vi "Begin.vi"(8 "error in":errorcluster) -> (0 "error out":errorcluster)   [LabVIEW 2018]
doc: "Called before other user functions, this VI is expected to open initial I/O refnums, load in file data, and do all program initialization. Notice that the <B>error out</B> terminal is simply used for data flow. Wiring it to other structures or subVIs ensures that this VI runs first."
uses:
  <vilib>/Rock Robotics/WPI/Joystick/WPI_JoystickDeviceEnum.ctl
  <vilib>/Rock Robotics/WPI/DriverStation/WPI_DriverStationRobotMode2.ctl
  <vilib>/Rock Robotics/SystemInterfaces/DIO/FPGA_DIOChannel.ctl
  <vilib>/Rock Robotics/WPI/Solenoid/WPI_SolenoidChannel.ctl
  <vilib>/Rock Robotics/WPI/ThirdParty/Phoenix-LabVIEW/Motor Controller/Controls/CTRE_Phoenix_MotorControl_NeutralMode.ctl
  Robot Global Data.vi
  <vilib>/Rock Robotics/Network Tables/NT Write String Array.vi
  <vilib>/Rock Robotics/WPI/Solenoid/WPI_SolenoidOpenDouble.vi
  <vilib>/Rock Robotics/WPI/RobotDrive/WPI_RobotDriveOpen2MotorWithExistingMotors.vi
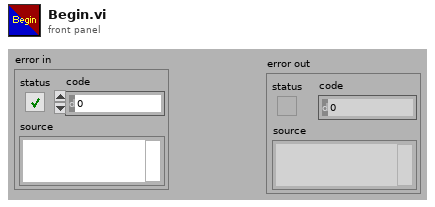
[diagram p1: front panel]
types:
  T1 = typedef "WPI_JoystickDeviceEnum.ctl" = enum16{"USB 0", "USB 1", "USB 2", "USB 3", "USB 4", "USB 5"}
  T2 = typedef "FPGA_DIOChannel.ctl" = enum8{"DIO 0", "DIO 1", "DIO 2", "DIO 3", "DIO 4", "DIO 5", "DIO 6", "DIO 7", "DIO 8", "DIO 9", "DIO MXP 0", "DIO MXP 1", "DIO MXP 2", "DIO MXP 3", "DIO MXP 4", "DIO MXP 5", "DIO MXP 6", "DIO MXP 7", "DIO MXP 8", "DIO MXP 9", "DIO MXP 10", "DIO MXP 11", "DIO MXP 12", "DIO MXP 13", "DIO MXP 14", "DIO MXP 15", "SPI Port CS1", "SPI Port CS2", "SPI Port CS3", "SPI Port MISO", "SPI Port MOSI", "Invalid"}
  T3 = typedef "WPI_SolenoidChannel.ctl" = enum8{"Solenoid 0", "Solenoid 1", "Solenoid 2", "Solenoid 3", "Solenoid 4", "Solenoid 5", "Solenoid 6", "Solenoid 7", "Invalid"}
  T4 = typedef "WPI_DriverStationRobotMode2.ctl" = enum16{"Autonomous Disabled", "Autonomous Enabled", "Teleop Disabled", "Teleop Enabled", "Disconnected", "Finish", "Test Disabled", "Test Enabled", "Emergency Stopped"}
  T5 = cluster{"proportional gain (Kc)":dbl, "integral time (Ti, min)":dbl, "derivative time (Td, min)":dbl}
  T6 = typedef "WPI_JoystickDevRef.ctl" = cluster{"Device":T1}
  T7 = typedef "CTRE_Phoenix_MotorControl_NeutralMode.ctl" = enum8{"EEPROMSetting", "Override to Coast", "Override to Brake"}
  T8 = cluster{"Yaw":dbl, "Roll":dbl, "Pitch":dbl, "Heading":dbl, "Fused Heading":dbl}
  T9 = typedef "WPI_MotorControlDeviceRef.ctl" = cluster{"DeviceStatus":errorcluster, "Type":T10, "PWM":cluster{"PWM Channel":T11, "DeadBand":T12}, "CAN":cluster{"Device Number":u8, "SetOutput VI Ref":variant, "GetOutput VI Ref":variant, "Enable VI Ref":variant, "Disable VI Ref":variant, "Data":variant}, "Invert":bool, "DIO PWM":cluster{"PWM \"Enable\" Channel":T11, "DIOChannel":T2, "PWM Rate":dbl}}
  T10 = typedef "WPI_MotorControlType.ctl" = enum16{"PWM", "CAN", "DIO PWM"}
  T11 = typedef "FPGA_DIOPWMChannel.ctl" = enum8{"PWM 0", "PWM 1", "PWM 2", "PWM 3", "PWM 4", "PWM 5", "PWM 6", "PWM 7", "PWM 8", "PWM 9", "PWM MXP 0", "PWM MXP 1", "PWM MXP 2", "PWM MXP 3", "PWM MXP 4", "PWM MXP 5", "PWM MXP 6", "PWM MXP 7", "PWM MXP 8", "PWM MXP 9", "Invalid"}
  T12 = typedef "WPI_PWMDeadband.ctl" = cluster{"Name":string, "maxPositivePwm":i32, "minPositivePwm":i32, "centerPwm":i32, "maxNegativePwm":i32, "minNegativePwm":i32, "angularRange":u16}
  T13 = typedef "WPI_RobotDriveDevRef.ctl" = cluster{"DevStatus":errorcluster, "Motors[]":T9[], "Square Inputs":bool, "Max Output":dbl}
  T14 = typedef "WPI_DigitalInputDevRef.ctl" = cluster{"DevStatus":errorcluster, "DIO Channel":T2}
  T15 = typedef "WPI_SolenoidDevRef.ctl" = cluster{"DevStatus":errorcluster, "Pneumatics Control Module":u8, "Forward Solenoid Channel":T3, "Reverse Solenoid Channel":T3}
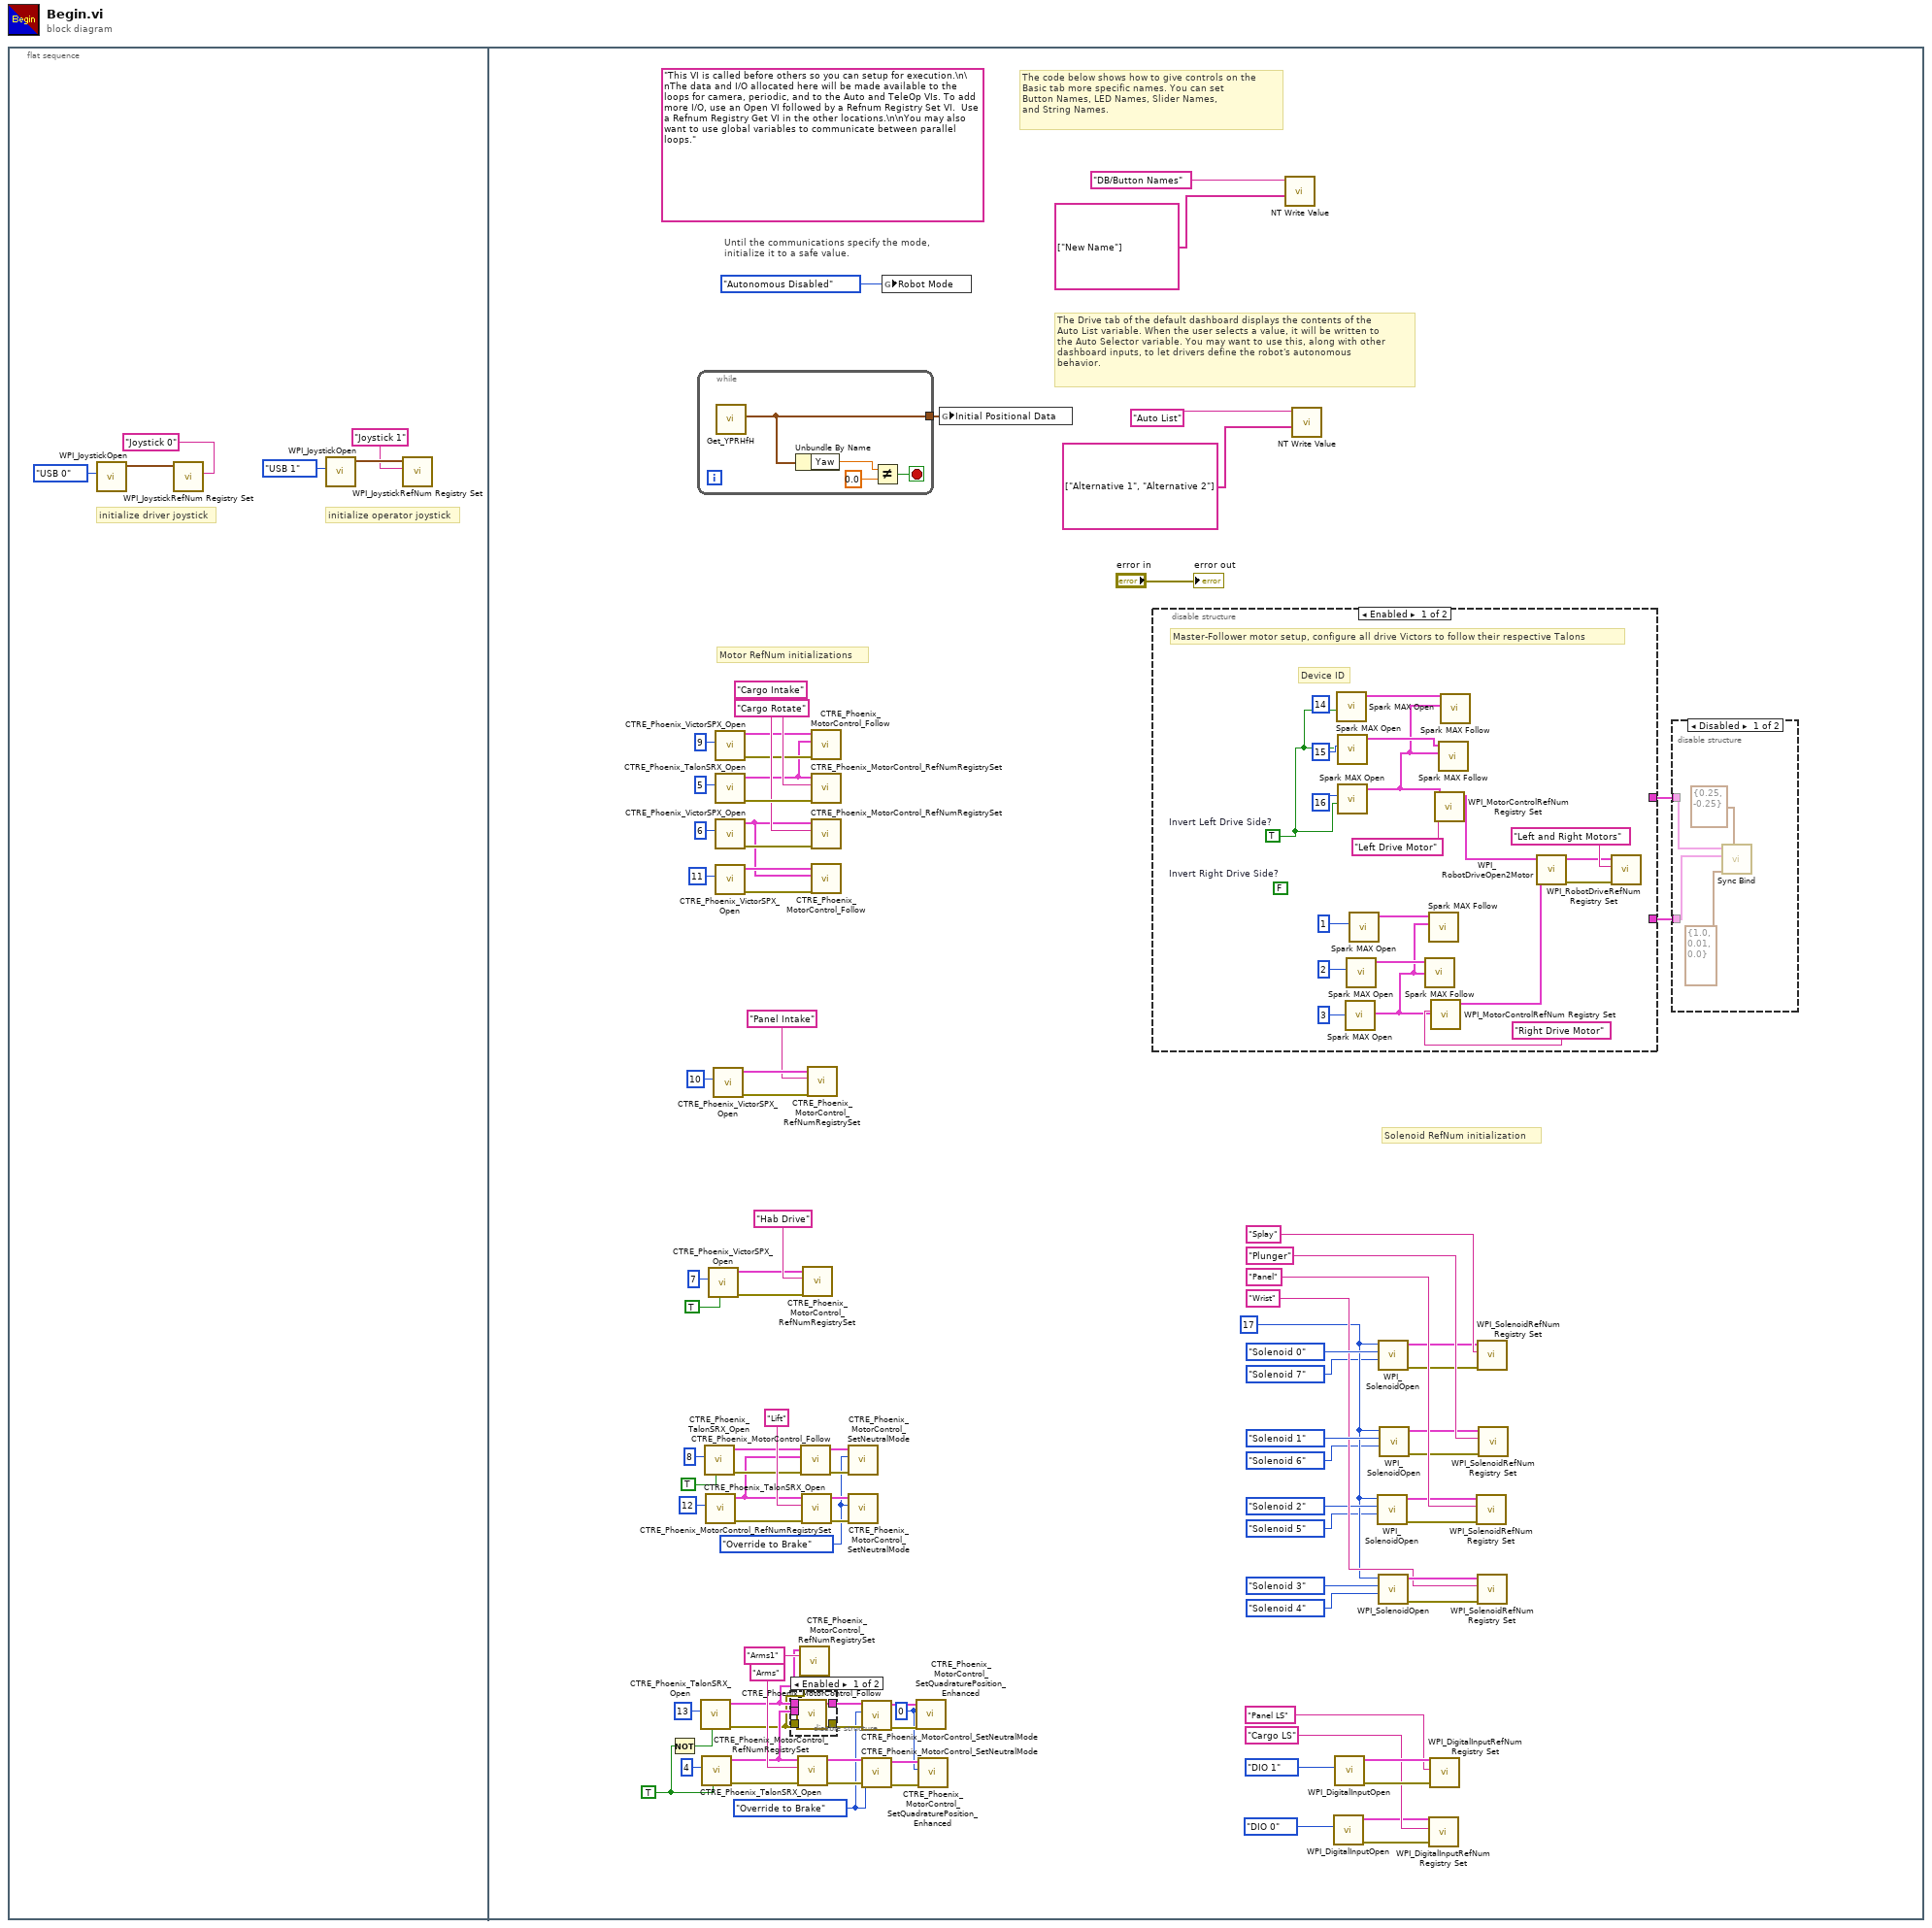
[diagram p0: block diagram]
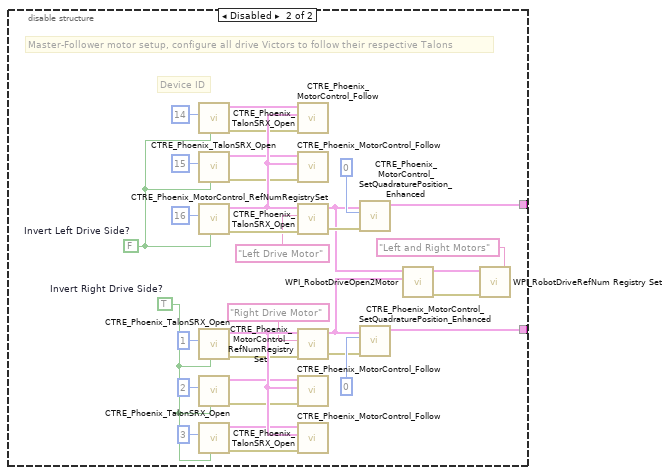
[diagram p4: hidden frame]
diagram:
  n1 = flat-sequence {
    frame #0 {
      # "initialize operator joystick"
      # "initialize driver joystick"
      n2 = call <vilib>:"WPI_JoystickOpen.vi"("JoystickDevice"=WPI_JoystickDeviceEnum."USB 0") -> ("JoystickDevRef"=w5:T6)  [unwired: 10 in]
      n3 = call <vilib>:"WPI_JoystickRefNum Registry Set.vi"("refnum name"="Joystick 0", "JoystickDevRef"=w5) -> ()  [unwired: 8 in, 2 out]
      n4 = call <vilib>:"WPI_JoystickOpen.vi"("JoystickDevice"=WPI_JoystickDeviceEnum."USB 1") -> ("JoystickDevRef"=w6:T6)  [unwired: 10 in]
      n5 = call <vilib>:"WPI_JoystickRefNum Registry Set.vi"("refnum name"="Joystick 1", "JoystickDevRef"=w6) -> ()  [unwired: 8 in, 2 out]
    }
    frame #1 {
      w8 = 0 ("New Position")
      w28 = u8 17 ("Pneumatics Control Module (0)")
      w34 = TRUE ("Invert")
      w36 = CTRE_Phoenix_MotorControl_NeutralMode."Override to Brake" ("Motor Control Neutral Mode")
      w42 = CTRE_Phoenix_MotorControl_NeutralMode."Override to Brake" ("Motor Control Neutral Mode")
      (unwired) "This VI is called before others so you can setup for execution.\n\nThe data and I/O allocated here will be made available to the loops for camera, periodic, and to the Auto and TeleOp VIs. To add more I/O, use an Open VI followed by a Refnum Registry Set VI.  Use a Refnum Registry Get VI in the other locations.\n\nYou may also want to use global variables to communicate between parallel loops."
      # "Motor RefNum initializations"
      # "Solenoid RefNum initialization"
      # "The Drive tab of the default dashboard displays the contents of the\nAuto List variable. When the user selects a value, it will be written to\nthe Auto Selector variable. You may want to use this, along with other\ndashboard inputs, to let drivers define the robot's autonomous\nbehavior."
      # "The code below shows how to give controls on the\nBasic tab more specific names. You can set\nButton Names, LED Names, Slider Names,\nand String Names."
      # "Until the communications specify the mode,\ninitialize it to a safe value."
      n6 = Not(x=w34) -> (.not. x?=w33:bool)
      n7 = while {
        tunnel: [w112] -> w27
        stop <- w113 stop-if-true
        n8 = call <vilib>:"Get_YPRHfH.vi"() -> ("YRPHfH"=w112:T8)  [unwired: 11 in]
        n9 = Unbundle By Name(w112) -> ("Yaw"=w114:dbl)
        n10 = Not Equal?(x=w114, y=0.0) -> (x != y?=w113:bool)
      }
      n11 = call <vilib>:"CTRE_Phoenix_TalonSRX_Open.vi"("Invert"=w33, "Device Number"=u8 13) -> ("error out"=w14:errorcluster, "CAN Talon SRX Ref"=w15:T9)  [unwired: 8 in]
      n12 = call <vilib>:"CTRE_Phoenix_TalonSRX_Open.vi"("Invert"=w34, "Device Number"=u8 4) -> ("error out"=w56:errorcluster, "CAN Talon SRX Ref"=w41:T9)  [unwired: 8 in]
      n13 = call <vilib>:"CTRE_Phoenix_TalonSRX_Open.vi"("Invert"=TRUE, "Device Number"=u8 8) -> ("error out"=w59:errorcluster, "CAN Talon SRX Ref"=w60:T9)  [unwired: 8 in]
      n14 = call <vilib>:"CTRE_Phoenix_TalonSRX_Open.vi"("Device Number"=u8 12) -> ("error out"=w58:errorcluster, "CAN Talon SRX Ref"=w57:T9)  [unwired: 9 in]
      n15 = call <vilib>:"CTRE_Phoenix_VictorSPX_Open.vi"("Invert"=TRUE, "Device Number"=u8 7) -> ("error out"=w50:errorcluster, "CAN Talon SRX Ref"=w49:T9)  [unwired: 8 in]
      n16 = call <vilib>:"CTRE_Phoenix_VictorSPX_Open.vi"("Device Number"=u8 10) -> ("error out"=w69:errorcluster, "CAN Talon SRX Ref"=w70:T9)  [unwired: 9 in]
      n17 = call <vilib>:"CTRE_Phoenix_VictorSPX_Open.vi"("Device Number"=u8 9) -> ("error out"=w18:errorcluster, "CAN Talon SRX Ref"=w19:T9)  [unwired: 9 in]
      n18 = call <vilib>:"CTRE_Phoenix_TalonSRX_Open.vi"("Device Number"=u8 5) -> ("error out"=w74:errorcluster, "CAN Talon SRX Ref"=w17:T9)  [unwired: 9 in]
      n19 = call <vilib>:"CTRE_Phoenix_VictorSPX_Open.vi"("Device Number"=u8 6) -> ("error out"=w73:errorcluster, "CAN Talon SRX Ref"=w46:T9)  [unwired: 9 in]
      n20 = call <vilib>:"CTRE_Phoenix_VictorSPX_Open.vi"("Device Number"=u8 11) -> ("error out"=w47:errorcluster, "CAN Talon SRX Ref"=w48:T9)  [unwired: 9 in]
      n21 = disable-structure shown="Enabled" {
        disable-tunnel: [w105 w107] -> w13
        disable-tunnel: [w104 w106] -> w45
        disable-tunnel: w41 -> [w103 _]
        disable-tunnel: w15 -> [w102 w107]
        disable-tunnel: w14 -> [w101 w106]
        frame Enabled {
          n22 = call <vilib>:"CTRE_Phoenix_MotorControl_Follow.vi"("error in (no error)"=w101, "Master Controller to Follow"=w103, "PhoenixMotorControlDevRef"=w102) -> ("error out"=w104:errorcluster, "PhoenixMotorControlDevRef"=w105:T9)  [unwired: 7 in]
        }
        frame Disabled {
        }
      }
      n23 = call <vilib>:"CTRE_Phoenix_MotorControl_RefNumRegistrySet.vi"("error in (no error)"=w56, "refnum name"="Arms", "PhoenixMotorControlDevRef"=w41) -> ("error out"=w44:errorcluster, "PhoenixMotorControlDevRef"=w43:T9)  [unwired: 7 in]
      n24 = call <vilib>:"CTRE_Phoenix_MotorControl_RefNumRegistrySet.vi"("error in (no error)"=w14, "refnum name"="Arms1", "PhoenixMotorControlDevRef"=w15) -> ()  [unwired: 7 in, 2 out]
      n25 = call <vilib>:"CTRE_Phoenix_MotorControl_Follow.vi"("error in (no error)"=w59, "Master Controller to Follow"=w57, "PhoenixMotorControlDevRef"=w60) -> ("error out"=w37:errorcluster, "PhoenixMotorControlDevRef"=w38:T9)  [unwired: 7 in]
      n26 = call <vilib>:"CTRE_Phoenix_MotorControl_RefNumRegistrySet.vi"("error in (no error)"=w58, "refnum name"="Lift", "PhoenixMotorControlDevRef"=w57) -> ("error out"=w40:errorcluster, "PhoenixMotorControlDevRef"=w39:T9)  [unwired: 7 in]
      n27 = call <vilib>:"CTRE_Phoenix_MotorControl_RefNumRegistrySet.vi"("error in (no error)"=w50, "refnum name"="Hab Drive", "PhoenixMotorControlDevRef"=w49) -> ()  [unwired: 7 in, 2 out]
      n28 = call <vilib>:"CTRE_Phoenix_MotorControl_RefNumRegistrySet.vi"("error in (no error)"=w69, "refnum name"="Panel Intake", "PhoenixMotorControlDevRef"=w70) -> ()  [unwired: 7 in, 2 out]
      n29 = call <vilib>:"CTRE_Phoenix_MotorControl_Follow.vi"("error in (no error)"=w18, "Master Controller to Follow"=w17, "PhoenixMotorControlDevRef"=w19) -> ()  [unwired: 7 in, 2 out]
      n30 = call <vilib>:"CTRE_Phoenix_MotorControl_RefNumRegistrySet.vi"("error in (no error)"=w74, "refnum name"="Cargo Rotate", "PhoenixMotorControlDevRef"=w17) -> ()  [unwired: 7 in, 2 out]
      n31 = call <vilib>:"CTRE_Phoenix_MotorControl_RefNumRegistrySet.vi"("error in (no error)"=w73, "refnum name"="Cargo Intake", "PhoenixMotorControlDevRef"=w46) -> ()  [unwired: 7 in, 2 out]
      n32 = call <vilib>:"CTRE_Phoenix_MotorControl_Follow.vi"("error in (no error)"=w47, "Master Controller to Follow"=w46, "PhoenixMotorControlDevRef"=w48) -> ()  [unwired: 7 in, 2 out]
      n33 = call <vilib>:"CTRE_Phoenix_MotorControl_SetNeutralMode.vi"("error in (no error)"=w37, "Motor Control Neutral Mode"=w36, "PhoenixMotorControlDevRef"=w38) -> ()  [unwired: 7 in, 2 out]
      n34 = call <vilib>:"CTRE_Phoenix_MotorControl_SetNeutralMode.vi"("error in (no error)"=w40, "Motor Control Neutral Mode"=w36, "PhoenixMotorControlDevRef"=w39) -> ()  [unwired: 7 in, 2 out]
      n35 = call <vilib>:"CTRE_Phoenix_MotorControl_SetNeutralMode.vi"("error in (no error)"=w45, "Motor Control Neutral Mode"=w42, "PhoenixMotorControlDevRef"=w13) -> ("error out"=w12:errorcluster, "PhoenixMotorControlDevRef"=w11:T9)  [unwired: 7 in]
      n36 = call <vilib>:"CTRE_Phoenix_MotorControl_SetNeutralMode.vi"("error in (no error)"=w44, "Motor Control Neutral Mode"=w42, "PhoenixMotorControlDevRef"=w43) -> ("error out"=w10:errorcluster, "PhoenixMotorControlDevRef"=w9:T9)  [unwired: 7 in]
      n37 = global write "Robot Global Data.vi" "Robot Mode"(WPI_DriverStationRobotMode2."Autonomous Disabled" ("Robot Mode")) -> ()
      n38 = call <vilib>:"CTRE_Phoenix_MotorControl_SetQuadraturePosition_Enhanced.vi"("error in (no error)"=w12, "New Position"=w8, "PhoenixMotorControlDevRef"=w11) -> ()  [unwired: 7 in, 2 out]
      n39 = call <vilib>:"CTRE_Phoenix_MotorControl_SetQuadraturePosition_Enhanced.vi"("error in (no error)"=w10, "New Position"=w8, "PhoenixMotorControlDevRef"=w9) -> ()  [unwired: 7 in, 2 out]
      n40 = global write "Robot Global Data.vi" "Initial Positional Data"(w27) -> ()
      n41 = disable-structure shown="Enabled" {
        disable-tunnel: [_ w136] -> w26
        disable-tunnel: [_ w135] -> w25
        frame Enabled {
          (unwired) u8 14 ("Device Number")
          w128 = TRUE  # Invert Left Drive Side?
          (unwired) FALSE  # Invert Right Drive Side?
          # "Master-Follower motor setup, configure all drive Victors to follow their respective Talons"
          # "Device ID"
          n42 = call <vilib>:"Spark MAX Open.vi"("Invert"=w128) -> ("MotorControlDeviceRef"=w131:T9)  [unwired: 9 in, 1 out]
          n43 = call <vilib>:"Spark MAX Open.vi"("Invert"=w128, "Device Number"=u8 15) -> ("MotorControlDeviceRef"=w127:T9)  [unwired: 8 in, 1 out]
          n44 = call <vilib>:"Spark MAX Open.vi"("Invert"=w128, "Device Number"=u8 16) -> ("MotorControlDeviceRef"=w126:T9)  [unwired: 8 in, 1 out]
          n45 = call <vilib>:"Spark MAX Open.vi"("Device Number"=u8 3) -> ("MotorControlDeviceRef"=w117:T9)  [unwired: 9 in, 1 out]
          n46 = call <vilib>:"Spark MAX Open.vi"("Device Number"=u8 2) -> ("MotorControlDeviceRef"=w119:T9)  [unwired: 9 in, 1 out]
          n47 = call <vilib>:"Spark MAX Open.vi"("Device Number"=u8 1) -> ("MotorControlDeviceRef"=w118:T9)  [unwired: 9 in, 1 out]
          n48 = call <vilib>:"Spark MAX Follow.vi"("Master Controller"=w117, "MotorControlDeviceRef"=w119) -> ()  [unwired: 8 in, 2 out]
          n49 = call <vilib>:"Spark MAX Follow.vi"("Master Controller"=w117, "MotorControlDeviceRef"=w118) -> ()  [unwired: 8 in, 2 out]
          n50 = call <vilib>:"WPI_MotorControlRefNum Registry Set.vi"("refnum name"="Right Drive Motor", "MotorControlDevRef"=w117) -> ("MotorControlDevRef"=w116:T9)  [unwired: 8 in, 1 out]
          n51 = call <vilib>:"WPI_MotorControlRefNum Registry Set.vi"("refnum name"="Left Drive Motor", "MotorControlDevRef"=w126) -> ("MotorControlDevRef"=w125:T9)  [unwired: 8 in, 1 out]
          n52 = call <vilib>:"Spark MAX Follow.vi"("Master Controller"=w126, "MotorControlDeviceRef"=w127) -> ()  [unwired: 8 in, 2 out]
          n53 = call <vilib>:"Spark MAX Follow.vi"("Master Controller"=w126, "MotorControlDeviceRef"=w131) -> ()  [unwired: 8 in, 2 out]
          n54 = call-poly <vilib>:"WPI_RobotDriveOpen2Motor.vi"("Right Motor Dev Ref"=w116, "Left Motor Dev Ref"=w125) -> ("error out"=w132:errorcluster, "RobotDriveDevRef"=w133:T13)  [unwired: 8 in]
          n55 = call <vilib>:"WPI_RobotDriveRefNum Registry Set.vi"("error in (no error)"=w132, "refnum name"="Left and Right Motors", "RobotDriveDevRef"=w133) -> ()  [unwired: 7 in, 2 out]
        }
        frame Disabled {
          w149 = FALSE  # Invert Left Drive Side?
          w150 = TRUE  # Invert Right Drive Side?
          # "Master-Follower motor setup, configure all drive Victors to follow their respective Talons"
          # "Device ID"
          n56 = call <vilib>:"CTRE_Phoenix_TalonSRX_Open.vi"("Invert"=w149, "Device Number"=u8 14) -> ("error out"=w162:errorcluster, "CAN Talon SRX Ref"=w163:T9)  [unwired: 8 in]
          n57 = call <vilib>:"CTRE_Phoenix_TalonSRX_Open.vi"("Invert"=w149, "Device Number"=u8 15) -> ("error out"=w161:errorcluster, "CAN Talon SRX Ref"=w164:T9)  [unwired: 8 in]
          n58 = call <vilib>:"CTRE_Phoenix_TalonSRX_Open.vi"("Invert"=w149, "Device Number"=u8 16) -> ("error out"=w154:errorcluster, "CAN Talon SRX Ref"=w165:T9)  [unwired: 8 in]
          n59 = call <vilib>:"CTRE_Phoenix_TalonSRX_Open.vi"("Invert"=w150, "Device Number"=u8 1) -> ("error out"=w155:errorcluster, "CAN Talon SRX Ref"=w160:T9)  [unwired: 8 in]
          n60 = call <vilib>:"CTRE_Phoenix_TalonSRX_Open.vi"("Invert"=w150, "Device Number"=u8 2) -> ("error out"=w156:errorcluster, "CAN Talon SRX Ref"=w157:T9)  [unwired: 8 in]
          n61 = call <vilib>:"CTRE_Phoenix_TalonSRX_Open.vi"("Invert"=w150, "Device Number"=u8 3) -> ("error out"=w159:errorcluster, "CAN Talon SRX Ref"=w158:T9)  [unwired: 8 in]
          n62 = call <vilib>:"CTRE_Phoenix_MotorControl_Follow.vi"("error in (no error)"=w162, "Master Controller to Follow"=w165, "PhoenixMotorControlDevRef"=w163) -> ()  [unwired: 7 in, 2 out]
          n63 = call <vilib>:"CTRE_Phoenix_MotorControl_Follow.vi"("error in (no error)"=w161, "Master Controller to Follow"=w165, "PhoenixMotorControlDevRef"=w164) -> ()  [unwired: 7 in, 2 out]
          n64 = call <vilib>:"CTRE_Phoenix_MotorControl_RefNumRegistrySet.vi"("error in (no error)"=w154, "refnum name"="Left Drive Motor", "PhoenixMotorControlDevRef"=w165) -> ("error out"=w138:errorcluster, "PhoenixMotorControlDevRef"=w137:T9)  [unwired: 7 in]
          n65 = call <vilib>:"CTRE_Phoenix_MotorControl_RefNumRegistrySet.vi"("error in (no error)"=w155, "refnum name"="Right Drive Motor", "PhoenixMotorControlDevRef"=w160) -> ("error out"=w139:errorcluster, "PhoenixMotorControlDevRef"=w140:T9)  [unwired: 7 in]
          n66 = call <vilib>:"CTRE_Phoenix_MotorControl_Follow.vi"("error in (no error)"=w156, "Master Controller to Follow"=w160, "PhoenixMotorControlDevRef"=w157) -> ()  [unwired: 7 in, 2 out]
          n67 = call <vilib>:"CTRE_Phoenix_MotorControl_Follow.vi"("error in (no error)"=w159, "Master Controller to Follow"=w160, "PhoenixMotorControlDevRef"=w158) -> ()  [unwired: 7 in, 2 out]
          n68 = call <vilib>:"CTRE_Phoenix_MotorControl_SetQuadraturePosition_Enhanced.vi"("error in (no error)"=w138, "New Position"=0, "PhoenixMotorControlDevRef"=w137) -> ("PhoenixMotorControlDevRef"=w136:T9)  [unwired: 7 in, 1 out]
          n69 = call <vilib>:"CTRE_Phoenix_MotorControl_SetQuadraturePosition_Enhanced.vi"("error in (no error)"=w139, "New Position"=0, "PhoenixMotorControlDevRef"=w140) -> ("PhoenixMotorControlDevRef"=w135:T9)  [unwired: 7 in, 1 out]
          n70 = call-poly <vilib>:"WPI_RobotDriveOpen2Motor.vi"("Right Motor Dev Ref"=w140, "Left Motor Dev Ref"=w137) -> ("error out"=w166:errorcluster, "RobotDriveDevRef"=w167:T13)  [unwired: 8 in]
          n71 = call <vilib>:"WPI_RobotDriveRefNum Registry Set.vi"("error in (no error)"=w166, "refnum name"="Left and Right Motors", "RobotDriveDevRef"=w167) -> ()  [unwired: 7 in, 2 out]
        }
      }
      n72 = call-poly <vilib>:"NT Write Value.vi"("String Array"=string[] ["New Name"], "Name"="DB/Button Names") -> ()  [unwired: 9 in, 1 out]
      n73 = call-poly <vilib>:"NT Write Value.vi"("String Array"=string[] ["Alternative 1", "Alternative 2"], "Name"="Auto List") -> ()  [unwired: 9 in, 1 out]
      n74 = call <vilib>:"WPI_DigitalInputOpen.vi"("DIO Channel"=FPGA_DIOChannel."DIO 0") -> ("error out"=w77:errorcluster, "DigitalInputDevRef"=w76:T14)  [unwired: 9 in]
      n75 = call <vilib>:"WPI_DigitalInputOpen.vi"("DIO Channel"=FPGA_DIOChannel."DIO 1") -> ("error out"=w92:errorcluster, "DigitalInputDevRef"=w93:T14)  [unwired: 9 in]
      n76 = call-poly <vilib>:"WPI_SolenoidOpen.vi"("Reverse Solenoid Channel"=WPI_SolenoidChannel."Solenoid 5" ("Solenoid Channel"), "Forward Solenoid Channel"=WPI_SolenoidChannel."Solenoid 2" ("Solenoid Channel"), "Pneumatics Control Module (0)"=w28) -> ("error out"=w84:errorcluster, "SolenoidDevRef"=w82:T15)  [unwired: 1 in, 6 out]
      n77 = call-poly <vilib>:"WPI_SolenoidOpen.vi"("Reverse Solenoid Channel"=WPI_SolenoidChannel."Solenoid 7" ("Solenoid Channel"), "Forward Solenoid Channel"=WPI_SolenoidChannel."Solenoid 0" ("Solenoid Channel"), "Pneumatics Control Module (0)"=w28) -> ("error out"=w31:errorcluster, "SolenoidDevRef"=w32:T15)  [unwired: 1 in, 6 out]
      n78 = call-poly <vilib>:"WPI_SolenoidOpen.vi"("Reverse Solenoid Channel"=WPI_SolenoidChannel."Solenoid 4" ("Solenoid Channel"), "Forward Solenoid Channel"=WPI_SolenoidChannel."Solenoid 3" ("Solenoid Channel"), "Pneumatics Control Module (0)"=w28) -> ("error out"=w85:errorcluster, "SolenoidDevRef"=w87:T15)  [unwired: 1 in, 6 out]
      n79 = call-poly <vilib>:"WPI_SolenoidOpen.vi"("Reverse Solenoid Channel"=WPI_SolenoidChannel."Solenoid 6" ("Solenoid Channel"), "Forward Solenoid Channel"=WPI_SolenoidChannel."Solenoid 1" ("Solenoid Channel"), "Pneumatics Control Module (0)"=w28) -> ("error out"=w30:errorcluster, "SolenoidDevRef"=w29:T15)  [unwired: 1 in, 6 out]
      n80 = call <vilib>:"WPI_DigitalInputRefNum Registry Set.vi"("error in (no error)"=w77, "refnum name"="Cargo LS", "DigitalInputDevRef"=w76) -> ()  [unwired: 7 in, 2 out]
      n81 = call <vilib>:"WPI_DigitalInputRefNum Registry Set.vi"("error in (no error)"=w92, "refnum name"="Panel LS", "DigitalInputDevRef"=w93) -> ()  [unwired: 7 in, 2 out]
      n82 = call <vilib>:"WPI_SolenoidRefNum Registry Set.vi"("error in (no error)"=w84, "refnum name"="Panel", "SolenoidDevRef"=w82) -> ()  [unwired: 7 in, 2 out]
      n83 = call <vilib>:"WPI_SolenoidRefNum Registry Set.vi"("error in (no error)"=w31, "refnum name"="Splay", "SolenoidDevRef"=w32) -> ()  [unwired: 7 in, 2 out]
      n84 = call <vilib>:"WPI_SolenoidRefNum Registry Set.vi"("error in (no error)"=w85, "refnum name"="Wrist", "SolenoidDevRef"=w87) -> ()  [unwired: 7 in, 2 out]
      n85 = call <vilib>:"WPI_SolenoidRefNum Registry Set.vi"("error in (no error)"=w30, "refnum name"="Plunger", "SolenoidDevRef"=w29) -> ()  [unwired: 7 in, 2 out]
      n86 = disable-structure shown="Disabled" {
        disable-tunnel: w26 -> [w111 _]
        disable-tunnel: w25 -> [w110 _]
        frame Disabled {
          n87 = call "Sync Bind.vi"("output range"=cluster{"output high":dbl, "output low":dbl} {"output high"=0.25, "output low"=-0.25}, "PID Constants"=T5 {"proportional gain (Kc)"=1.0, "integral time (Ti, min)"=0.01, "derivative time (Td, min)"=0.0}, "SlaveDevRef"=w110, "MasterDevRef"=w111) -> ()  [unwired: 8 in]
        }
        frame Enabled {
        }
      }
      "error out" <- "error in"
    }
  }
